vi "clone.vi"(0 "reference":refnum<class "CallNode.lvclass">, 5 "error in (no error)":errorcluster) -> (14 "reference out":refnum<class "CallNode.lvclass">, 15 "clonedCallNode":refnum<class "AbstractNode.lvclass">, 19 "error out":errorcluster)   [LabVIEW 2012, in "CallNode.lvclass"]
doc: "clone"
uses:
  <resource>/Framework/Providers/Open_GDS/UML/CallNode_class/CallNode.lvclass
  <resource>/Framework/Providers/Open_GDS/UML/AbstractNode_class/AbstractNode.lvclass
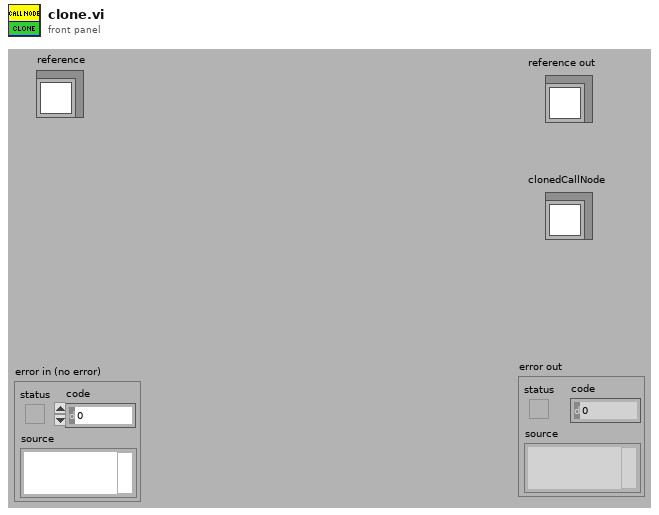
[diagram p1: front panel]
types:
  T1 = typedef "CallNode.lvclass/ObjectAttributes.ctl" = cluster{"Base class":T2, "objectCallNodeRef":refnum<class "AbstractNode.lvclass">, "signaled":bool, "openBottom":bool, "DEFAULT_WIDTH":i32, "DEFAULT_HEIGHT":i32, "CALL_YGAP":i32}
  T2 = typedef "RectangularNode.lvclass/ObjectAttributes.ctl" = cluster{"Base class":T3, "bounds":T4}
  T3 = typedef "AbstractNode.lvclass/ObjectAttributes.ctl" = cluster{"parent":refnum<class "AbstractNode.lvclass">, "children":refnum<class "AbstractNode.lvclass">[], "Hidden":bool}
  T4 = typedef "Rectangle Rectangle2D.ctl" = cluster{"x":dbl, "y":dbl, "width":dbl, "height":dbl}
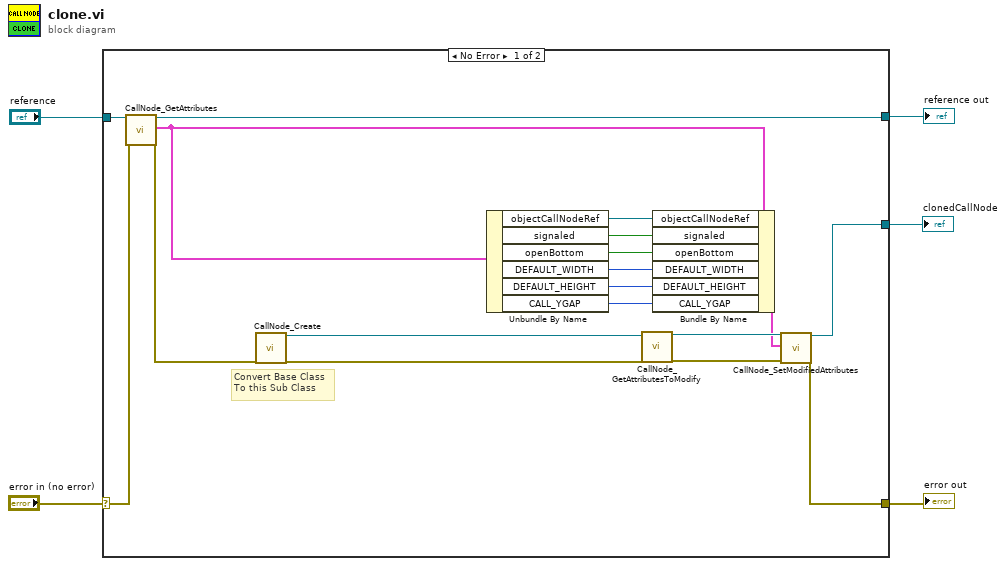
[diagram p0: block diagram]
diagram:
  n1 = case shown="No Error" "error in (no error)" {
    selector: "error in (no error)" -> [w23 w24]
    tunnel: "reference" -> [w22 w25]
    tunnel: [w11 w24] -> w3
    tunnel: [w7 w25] -> w2
    tunnel: [w12 _] -> w1
    frame No Error {
      # "Convert Base Class\nTo this Sub Class"
      n2 = call <resource>:"CallNode_GetAttributes.vi"("reference in"=w22, "error in (no error)"=w23) -> ("reference out"=w7:refnum<class "CallNode.lvclass">, "Attributes"=w9:T1, "error out"=w8:errorcluster)  [unwired: 15 out]
      n3 = call <resource>:"CallNode_Create.vi"("error in (no error)"=w8) -> ("reference out"=w6:refnum<class "CallNode.lvclass">, "error out"=w10:errorcluster)  [unwired: 16 in, 1 out]
      n4 = Unbundle By Name(w9) -> ("objectCallNodeRef"=w18:refnum<class "AbstractNode.lvclass">, "signaled"=w17:bool, "openBottom"=w16:bool, "DEFAULT_WIDTH"=w15:i32, "DEFAULT_HEIGHT"=w14:i32, "CALL_YGAP"=w13:i32)
      n5 = call <resource>:"CallNode_GetAttributesToModify.vi"("reference in"=w6, "error in (no error)"=w10) -> ("reference out"=w21:refnum<class "CallNode.lvclass">, "error out"=w20:errorcluster)  [unwired: 1 in, 15 out]
      n6 = Bundle By Name(cluster=w9, "objectCallNodeRef"=w18, "signaled"=w17, "openBottom"=w16, "DEFAULT_WIDTH"=w15, "DEFAULT_HEIGHT"=w14, "CALL_YGAP"=w13) -> (w19:T1)
      n7 = call <resource>:"CallNode_SetModifiedAttributes.vi"("reference in"=w21, "Attributes"=w19, "error in (no error)"=w20) -> ("reference out"=w12:refnum<class "CallNode.lvclass">, "error out"=w11:errorcluster)  [unwired: 3 in, 12 out]
    }
    frame Error {
    }
  }
  "reference out" <- w2
  "error out" <- w3
  "clonedCallNode" <- w1
